vi "BRig_dataMTrig_CueLed_T.vi"() -> (2 "output_CueLed_T":i32)   [LabVIEW 2014]
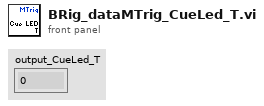
[diagram p1: front panel]
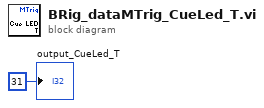
[diagram p0: block diagram]
diagram:
  "output_CueLed_T" <- 31 ("output_iBlock")
